vi "area (SubVI).vi"(8 "error in (no error)":errorcluster, 11 "Data":T1) -> (0 "error out":errorcluster, 3 "Numeric":dbl)   [LabVIEW 2023]
uses:
  #typedef_data.ctl
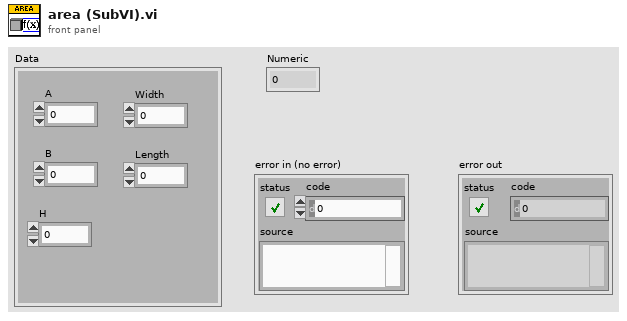
[diagram p1: front panel]
types:
  T1 = typedef "#typedef_data.ctl" = cluster{"A":dbl, "B":dbl, "H":dbl, "Width":dbl, "Length":dbl}
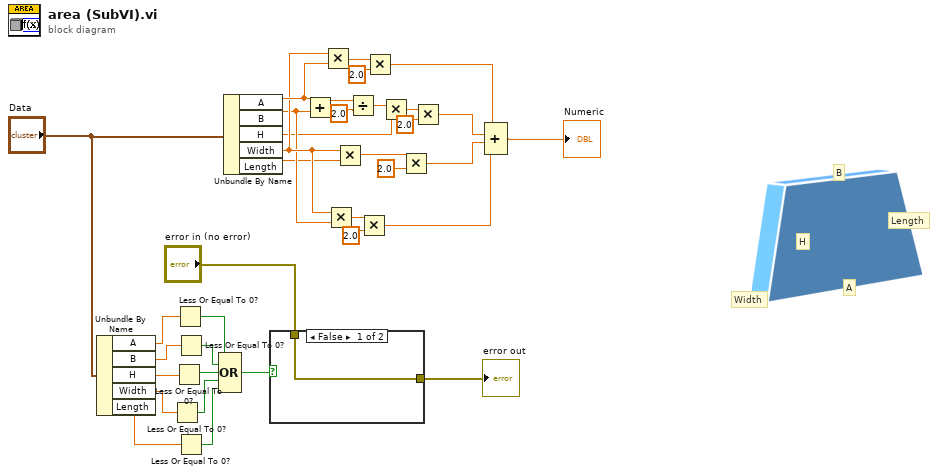
[diagram p0: block diagram]
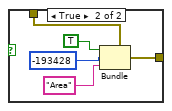
[diagram p2: hidden frame]
diagram:
  # "Length"
  # "Width"
  # "H"
  # "B"
  # "A"
  n1 = Unbundle By Name("Data") -> ("A"=w13:dbl, "B"=w12:dbl, "H"=w11:dbl, "Width"=w10:dbl, "Length"=w9:dbl)
  n2 = Less Or Equal To 0?(x=w10) -> (x <= 0?=w7:bool)
  n3 = Less Or Equal To 0?(x=w11) -> (x <= 0?=w6:bool)
  n4 = Less Or Equal To 0?(x=w13) -> (x <= 0?=w4:bool)
  n5 = Less Or Equal To 0?(x=w12) -> (x <= 0?=w5:bool)
  n6 = Less Or Equal To 0?(x=w9) -> (x <= 0?=w8:bool)
  n7 = Compound Arithmetic op=OR(w4, w5, w6, w7, w8) -> (w3:bool)
  n8 = Unbundle By Name("Data") -> ("A"=w30:dbl, "B"=w28:dbl, "H"=w18:dbl, "Width"=w29:dbl, "Length"=w19:dbl)
  n9 = case shown="False" w3 {
    tunnel: "error in (no error)" -> [w36 w41]
    tunnel: [w36 w37] -> w1
    frame False {
    }
    frame True {
      n10 = Bundle(cluster=w41, "status"=TRUE, "code"=-193428, "source"="Area") -> (w37:errorcluster)
    }
  }
  "error out" <- w1
  n11 = Add(x=w30, y=w28) -> (x+y=w16:dbl)
  n12 = Multiply(x=w29, y=w30) -> (x*y=w25:dbl)
  n13 = Multiply(x=w29, y=w28) -> (x*y=w27:dbl)
  n14 = Multiply(x=w29, y=w19) -> (x*y=w23:dbl)
  n15 = Divide(x=w16, y=2.0) -> (x/y=w17:dbl)
  n16 = Multiply(x=w27, y=2.0) -> (x*y=w34:dbl)
  n17 = Multiply(x=w25, y=2.0) -> (x*y=w33:dbl)
  n18 = Multiply(x=w17, y=w18) -> (x*y=w20:dbl)
  n19 = Multiply(x=w23, y=2.0) -> (x*y=w31:dbl)
  n20 = Multiply(x=w20, y=2.0) -> (x*y=w32:dbl)
  n21 = Compound Arithmetic op=ADD(w33, w32, w31, w34) -> (→"Numeric":dbl)
